vi "Trigger Controls New.vi"() -> ()   [LabVIEW 2012]
panel:
  in  "Tab Control":enum32{"CO", "AD"}(tab)=enum."AD"
  in  "High CO2 Forces":T1={"Main 1"=TRUE, "Main 2"=TRUE, "Recirc  3"=FALSE, "Boost A 7"=TRUE, "Recirc  9"=FALSE, "Scrub 4"=TRUE, "Scrub 10"=TRUE, "O2 5"=FALSE, "Vent 6"=TRUE, "Boost A 8"=TRUE, "Vent 11"=TRUE, "Boost B 12"=TRUE, "Boost B 13"=TRUE, "Recirc 14"=FALSE, "Scrub 15"=TRUE, "Vent 16"=TRUE, "Main 17"=TRUE, "Boost A 18"=TRUE, "Boost B 19"=TRUE, "Boost F 20"=TRUE, "Vent 2 21"=TRUE}
  in  "Run C1":T2={"Main 1"=inf, "Main 2"=inf, "Recirc  3"=9000.0, "Boost A 7"=3400.0, "Recirc  9"=9000.0, "Scrub 4"=8800.0, "Scrub 10"=8800.0, "O2 5"=9600.0, "Vent 6"=9200.0, "Boost A 8"=3400.0, "Vent 11"=9200.0, "Boost B 12"=1800.0, "Boost B 13"=1800.0, "Recirc 14"=9000.0, "Scrub 15"=8800.0, "Vent 16"=9200.0, "Main 17"=inf, "Boost A 18"=3400.0, "Boost B 19"=1800.0, "Boost F 20"=7000.0, "Vent 2 21"=9200.0}
  in  "Run C2":T2={"Main 1"=inf, "Main 2"=inf, "Recirc  3"=8800.0, "Boost A 7"=3000.0, "Recirc  9"=8800.0, "Scrub 4"=8600.0, "Scrub 10"=8600.0, "O2 5"=9600.0, "Vent 6"=9000.0, "Boost A 8"=3000.0, "Vent 11"=9000.0, "Boost B 12"=1400.0, "Boost B 13"=1400.0, "Recirc 14"=8800.0, "Scrub 15"=8600.0, "Vent 16"=9000.0, "Main 17"=inf, "Boost A 18"=3000.0, "Boost B 19"=1400.0, "Boost F 20"=6600.0, "Vent 2 21"=9000.0}
  in  "Hold C3":T2={"Main 1"=1800.0, "Main 2"=1800.0, "Recirc  3"=9000.0, "Boost A 7"=3400.0, "Recirc  9"=9000.0, "Scrub 4"=8800.0, "Scrub 10"=8800.0, "O2 5"=9600.0, "Vent 6"=9200.0, "Boost A 8"=3400.0, "Vent 11"=9200.0, "Boost B 12"=1800.0, "Boost B 13"=1800.0, "Recirc 14"=9000.0, "Scrub 15"=8800.0, "Vent 16"=9200.0, "Main 17"=inf, "Boost A 18"=3400.0, "Boost B 19"=1800.0, "Boost F 20"=7000.0, "Vent 2 21"=9200.0}
  in  "Hold C4":T2={"Main 1"=inf, "Main 2"=inf, "Recirc  3"=8800.0, "Boost A 7"=3000.0, "Recirc  9"=8800.0, "Scrub 4"=8600.0, "Scrub 10"=8600.0, "O2 5"=9600.0, "Vent 6"=9000.0, "Boost A 8"=3000.0, "Vent 11"=9000.0, "Boost B 12"=1400.0, "Boost B 13"=1400.0, "Recirc 14"=8800.0, "Scrub 15"=8600.0, "Vent 16"=9000.0, "Main 17"=inf, "Boost A 18"=3000.0, "Boost B 19"=1400.0, "Boost F 20"=6600.0, "Vent 2 21"=9000.0}
  in  "Hold A4":T2={"Main 1"=-150.0, "Main 2"=-150.0, "Recirc  3"=-30.0, "Boost A 7"=-250.0, "Recirc  9"=-30.0, "Scrub 4"=inf, "Scrub 10"=inf, "O2 5"=80.0, "Vent 6"=15.0, "Boost A 8"=-250.0, "Vent 11"=15.0, "Boost B 12"=-300.0, "Boost B 13"=-300.0, "Recirc 14"=-30.0, "Scrub 15"=inf, "Vent 16"=15.0, "Main 17"=-150.0, "Boost A 18"=-250.0, "Boost B 19"=-300.0, "Boost F 20"=-300.0, "Vent 2 21"=650.0}
  in  "Hold A3":T2={"Main 1"=0.0, "Main 2"=0.0, "Recirc  3"=50.0, "Boost A 7"=-150.0, "Recirc  9"=50.0, "Scrub 4"=inf, "Scrub 10"=inf, "O2 5"=150.0, "Vent 6"=60.0, "Boost A 8"=-150.0, "Vent 11"=60.0, "Boost B 12"=-200.0, "Boost B 13"=-200.0, "Recirc 14"=50.0, "Scrub 15"=inf, "Vent 16"=60.0, "Main 17"=0.0, "Boost A 18"=-150.0, "Boost B 19"=-200.0, "Boost F 20"=-200.0, "Vent 2 21"=700.0}
  in  "Run A1":T2={"Main 1"=-inf, "Main 2"=-inf, "Recirc  3"=-30.0, "Boost A 7"=-80.0, "Recirc  9"=-30.0, "Scrub 4"=inf, "Scrub 10"=inf, "O2 5"=80.0, "Vent 6"=15.0, "Boost A 8"=-80.0, "Vent 11"=15.0, "Boost B 12"=-50.0, "Boost B 13"=-50.0, "Recirc 14"=-30.0, "Scrub 15"=inf, "Vent 16"=15.0, "Main 17"=-inf, "Boost A 18"=0.0, "Boost B 19"=-50.0, "Boost F 20"=-80.0, "Vent 2 21"=650.0}
  in  "High AD Diff":T1={"Main 1"=FALSE, "Main 2"=FALSE, "Recirc  3"=FALSE, "Boost A 7"=FALSE, "Recirc  9"=FALSE, "Scrub 4"=FALSE, "Scrub 10"=TRUE, "O2 5"=FALSE, "Vent 6"=TRUE, "Boost A 8"=TRUE, "Vent 11"=TRUE, "Boost B 12"=TRUE, "Boost B 13"=TRUE, "Recirc 14"=FALSE, "Scrub 15"=TRUE, "Vent 16"=TRUE, "Main 17"=TRUE, "Boost A 18"=TRUE, "Boost B 19"=TRUE, "Boost F 20"=TRUE, "Vent 2 21"=TRUE}
  in  "Delay S":T2={"Main 1"=30.0, "Main 2"=30.0, "Recirc  3"=1.0, "Boost A 7"=30.0, "Recirc  9"=1.0, "Scrub 4"=1.0, "Scrub 10"=1.0, "O2 5"=1.0, "Vent 6"=1.0, "Boost A 8"=30.0, "Vent 11"=1.0, "Boost B 12"=30.0, "Boost B 13"=30.0, "Recirc 14"=1.0, "Scrub 15"=1.0, "Vent 16"=1.0, "Main 17"=30.0, "Boost A 18"=30.0, "Boost B 19"=30.0, "Boost F 20"=30.0, "Vent 2 21"=1.0}
  in  "Run A1":T2={"Main 1"=-inf, "Main 2"=-inf, "Recirc  3"=50.0, "Boost A 7"=0.0, "Recirc  9"=50.0, "Scrub 4"=inf, "Scrub 10"=inf, "O2 5"=150.0, "Vent 6"=60.0, "Boost A 8"=0.0, "Vent 11"=60.0, "Boost B 12"=15.0, "Boost B 13"=15.0, "Recirc 14"=50.0, "Scrub 15"=inf, "Vent 16"=60.0, "Main 17"=-inf, "Boost A 18"=0.0, "Boost B 19"=15.0, "Boost F 20"=0.0, "Vent 2 21"=700.0}
  in  "Alt Dif M":dbl(slide) scale=-1000.0..1000.0
  in  "CO2 ppm":dbl(slide) scale=0.0..10000.0 scale format="%#.0f"
  in  "Mode":enum16{"Run", "Hold", "Off"}(ring)
  out "Trigger":T1
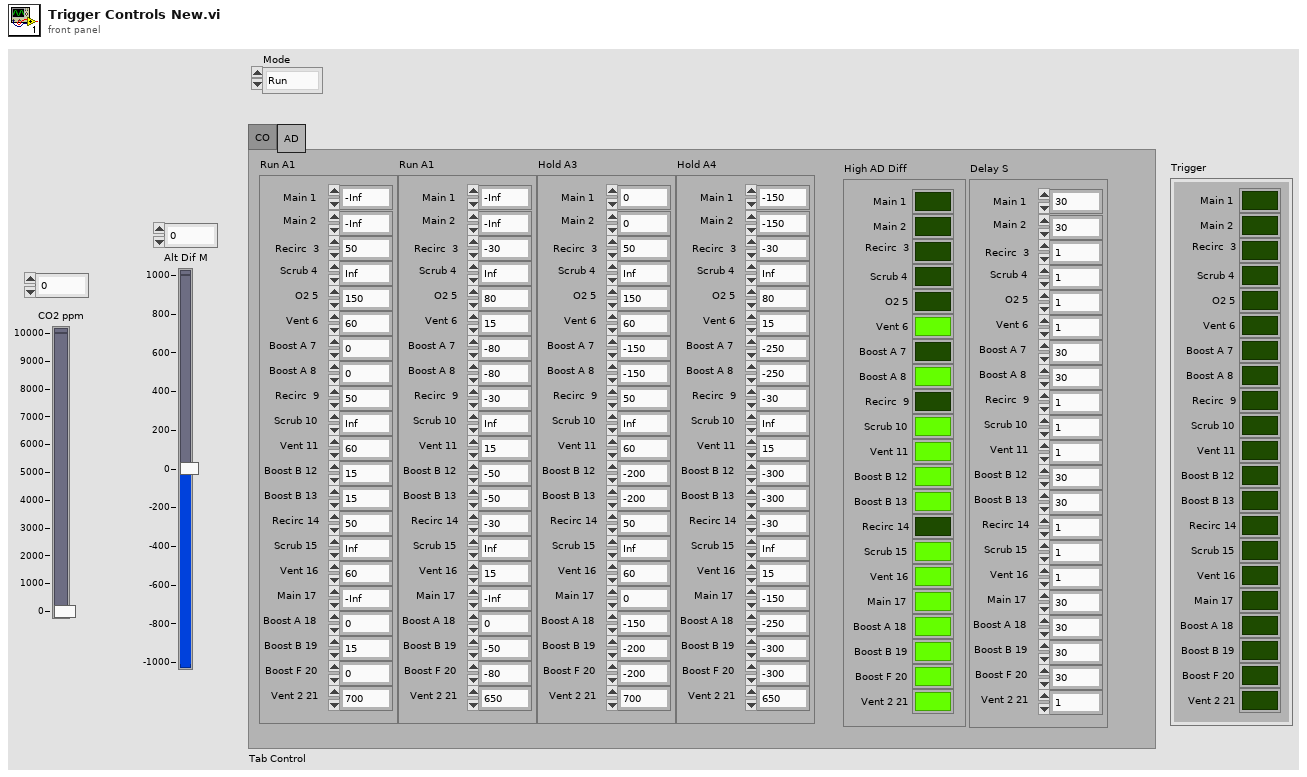
[diagram p1: front panel]
types:
  T1 = cluster{"Main 1":bool, "Main 2":bool, "Recirc  3":bool, "Boost A 7":bool, "Recirc  9":bool, "Scrub 4":bool, "Scrub 10":bool, "O2 5":bool, "Vent 6":bool, "Boost A 8":bool, "Vent 11":bool, "Boost B 12":bool, "Boost B 13":bool, "Recirc 14":bool, "Scrub 15":bool, "Vent 16":bool, "Main 17":bool, "Boost A 18":bool, "Boost B 19":bool, "Boost F 20":bool, "Vent 2 21":bool}
  T2 = cluster{"Main 1":dbl, "Main 2":dbl, "Recirc  3":dbl, "Boost A 7":dbl, "Recirc  9":dbl, "Scrub 4":dbl, "Scrub 10":dbl, "O2 5":dbl, "Vent 6":dbl, "Boost A 8":dbl, "Vent 11":dbl, "Boost B 12":dbl, "Boost B 13":dbl, "Recirc 14":dbl, "Scrub 15":dbl, "Vent 16":dbl, "Main 17":dbl, "Boost A 18":dbl, "Boost B 19":dbl, "Boost F 20":dbl, "Vent 2 21":dbl}
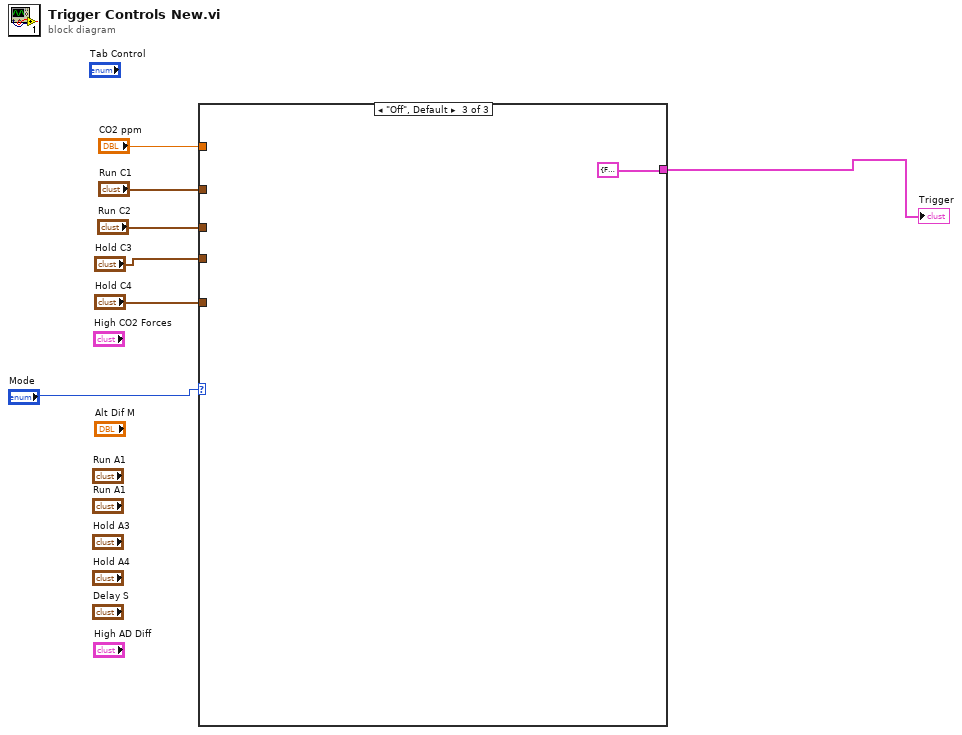
[diagram p0: block diagram]
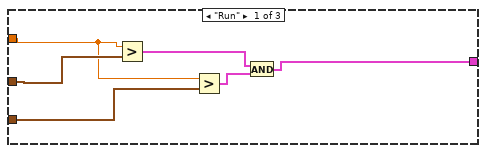
[diagram p2: hidden frame]
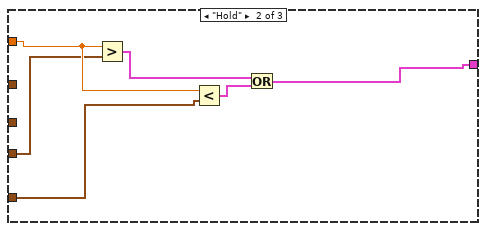
[diagram p3: hidden frame]
diagram:
  n1 = case shown="\"Off\", Default" "Mode" {
    tunnel: "CO2 ppm" -> [w9 w18 _]
    tunnel: "Run C1" -> [w10 _ _]
    tunnel: [w11 w17 T1 {"Main 1"=FALSE, "Main 2"=FALSE, "Recirc  3"=FALSE, "Boost A 7"=FALSE, "Recirc  9"=FALSE, "Scrub 4"=FALSE, "Scrub 10"=FALSE, "O2 5"=FALSE, "Vent 6"=FALSE, "Boost A 8"=FALSE, "Vent 11"=FALSE, "Boost B 12"=FALSE, "Boost B 13"=FALSE, "Recirc 14"=FALSE, "Scrub 15"=FALSE, "Vent 16"=FALSE, "Main 17"=FALSE, "Boost A 18"=FALSE, "Boost B 19"=FALSE, "Boost F 20"=FALSE, "Vent 2 21"=FALSE}] -> w4
    tunnel: "Run C2" -> [w8 _ _]
    tunnel: "Hold C3" -> [_ w15 _]
    tunnel: "Hold C4" -> [_ w14 _]
    frame "Run" {
      n2 = Greater?(x=w9, y=w10) -> (0:w13:T1)
      n3 = Greater?(x=w9, y=w8) -> (0:w12:T1)
      n4 = And(x=w13, y=w12) -> (x .and. y?=w11:T1)
    }
    frame "Hold" {
      n5 = Greater?(x=w18, y=w15) -> (0:w16:T1)
      n6 = Less?(x=w18, y=w14) -> (x < y?=w19:T1)
      n7 = Or(x=w16, y=w19) -> (x .or. y?=w17:T1)
    }
    frame "Off", Default {
    }
  }
  "Trigger" <- w4
